vi "Create Disconnect Messages.vi"(8 "error in (no error)":errorcluster, 11 "Engine Data in":T2) -> (0 "error out":errorcluster, 2 "Disconnect Messages":T1[](array[typedef]), 3 "Engine Data out":T2)   [LabVIEW 2017, in "Routing and Faulting Engine.lvlib"]
uses:
  Routing and Faulting Engine.lvlib
  Engine Data.ctl
  Includes/CDMessaging.lvlibp/Producer/Abstract Producer/Abstract Producer.lvclass
  Shared/Compiled.Settings.ctl
  Shared/Communication Configuration.ctl
  Shared/Routing and Faulting Configuration.ctl
  Shared/Routing Channel Configuration.ctl
  Shared/Value-Connections Map.ctl
  Shared/Connection.ctl
  Shared/Alias Mapping.ctl
  Shared/FIFO Indices.ctl
  Device Inputs.ctl
  Device Outputs.ctl
  Producer Message.ctl
  Includes/CDMessaging.lvlibp/Message/Abstract Message/Abstract Message.lvclass
  Shared/Routing and Faulting Shared.lvlib
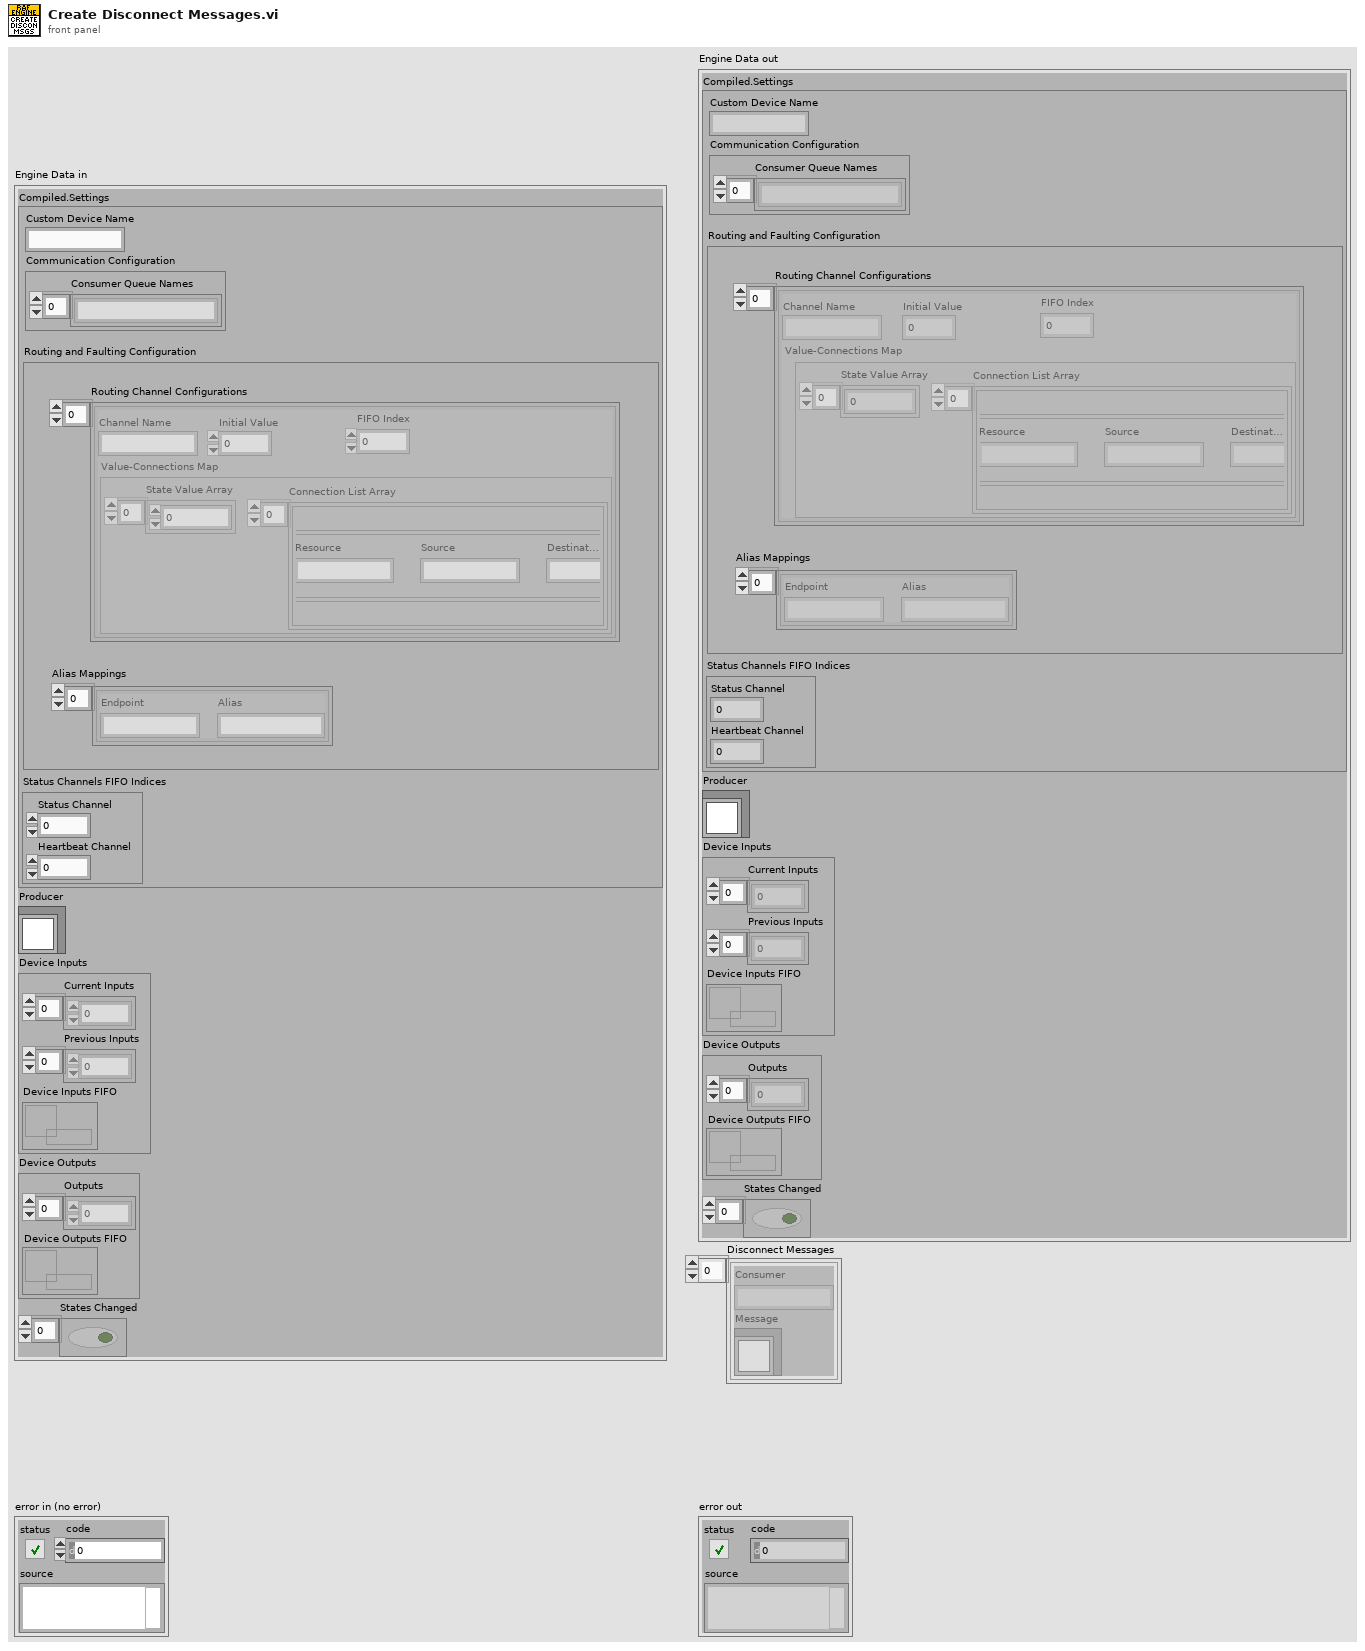
[diagram p1: front panel]
types:
  T1 = typedef "Routing and Faulting Engine.lvlib/Producer Message.ctl" = cluster{"Consumer":string, "Message":refnum<class "Abstract Message.lvclass">}
  T2 = typedef "Routing and Faulting Engine.lvlib/Engine Data.ctl" = cluster{"Compiled.Settings":T3, "Producer":refnum<class "Abstract Producer.lvclass">, "Device Inputs":T11, "Device Outputs":T12, "States Changed":bool[]}
  T3 = typedef "Routing and Faulting Shared.lvlib/Compiled.Settings.ctl" = cluster{"Custom Device Name":string, "Communication Configuration":T4, "Routing and Faulting Configuration":T5, "Status Channels FIFO Indices":T10}
  T4 = typedef "Routing and Faulting Shared.lvlib/Communication Configuration.ctl" = cluster{"Consumer Queue Names":string[]}
  T5 = typedef "Routing and Faulting Shared.lvlib/Routing and Faulting Configuration.ctl" = cluster{"Routing Channel Configurations":T6[], "Alias Mappings":T9[]}
  T6 = typedef "Routing and Faulting Shared.lvlib/Routing Channel Configuration.ctl" = cluster{"Channel Name":string, "Initial Value":dbl, "FIFO Index":i32, "Value-Connections Map":T7}
  T7 = typedef "Routing and Faulting Shared.lvlib/Value-Connections Map.ctl" = cluster{"State Value Array":i32[], "Connection List Array":cluster{"Connection List":T8[]}[]}
  T8 = typedef "Routing and Faulting Shared.lvlib/Connection.ctl" = cluster{"Resource":string, "Source":string, "Destination":string}
  T9 = typedef "Routing and Faulting Shared.lvlib/Alias Mapping.ctl" = cluster{"Endpoint":string, "Alias":string}
  T10 = typedef "Routing and Faulting Shared.lvlib/FIFO Indices.ctl" = cluster{"Status Channel":i32, "Heartbeat Channel":i32}
  T11 = typedef "Routing and Faulting Engine.lvlib/Device Inputs.ctl" = cluster{"Current Inputs":dbl[], "Previous Inputs":dbl[], "Device Inputs FIFO":refnum<k33>}
  T12 = typedef "Routing and Faulting Engine.lvlib/Device Outputs.ctl" = cluster{"Outputs":dbl[], "Device Outputs FIFO":refnum<k33>}
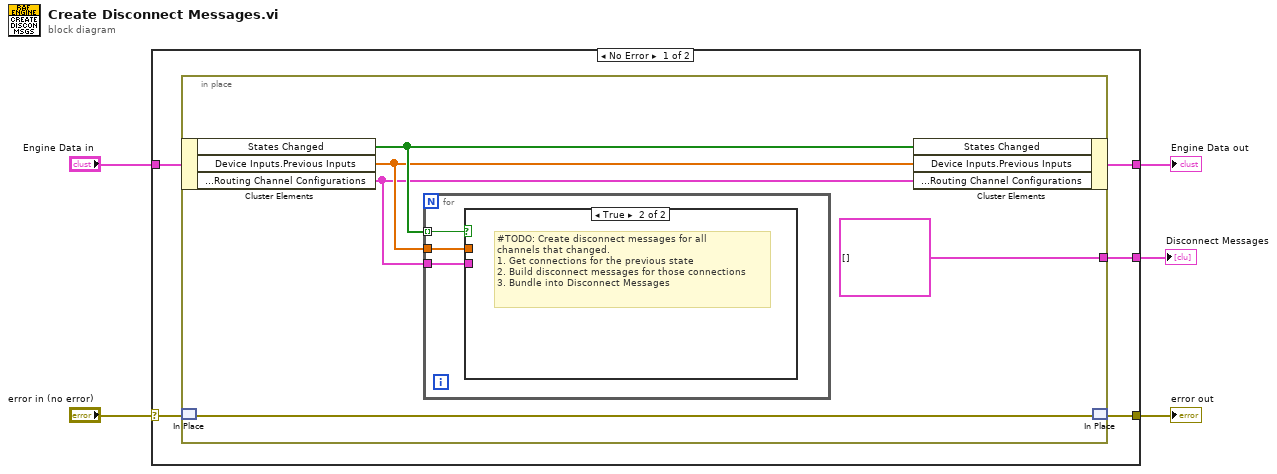
[diagram p0: block diagram]
diagram:
  n1 = case shown="No Error" "error in (no error)" {
    selector: "error in (no error)" -> [w10 w20]
    tunnel: "Engine Data in" -> [w8 w19]
    tunnel: [w9 w20] -> w3
    tunnel: [w7 w19] -> w2
    tunnel: [w6 _] -> w1
    frame No Error {
      n2 = in-place {
        in-place-border: [T1[] [] ("Disconnect Messages")] -> w6
        n3 = in-place-cluster #1(w8) -> ("States Changed"=w14:bool[], "Device Inputs.Previous Inputs"=w13:dbl[], "Compiled.Settings.Routing and Faulting Configuration.Routing Channel Configurations"=w12:T6[])
        n4 = in-place-match #2(w10) -> (w15:errorcluster)
        n5 = for {
          tunnel: w14 -> [w18] mode=indexing
          tunnel: w12 -> [w17]
          tunnel: w13 -> [w16]
          n6 = case shown="True" w18 {
            tunnel: w17 -> [_ _]
            tunnel: w16 -> [_ _]
            frame False {
              # "State didn't change. Do nothing"
            }
            frame True {
              # "#TODO: Create disconnect messages for all\nchannels that changed.\n1. Get connections for the previous state\n2. Build disconnect messages for those connections\n3. Bundle into Disconnect Messages"
            }
          }
        }
        n7 = in-place-cluster #1("States Changed"=w14, "Device Inputs.Previous Inputs"=w13, "Compiled.Settings.Routing and Faulting Configuration.Routing Channel Configurations"=w12) -> (w7:T2)
        n8 = in-place-match #2(w15) -> (w9:errorcluster)
      }
    }
    frame Error {
    }
  }
  "Engine Data out" <- w2
  "error out" <- w3
  "Disconnect Messages" <- w1
